vi "CRYWait Graph Close.vi"(10 "vi reference":refnum<vi>) -> ()   [LabVIEW 2013]
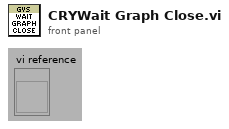
[diagram p1: front panel]
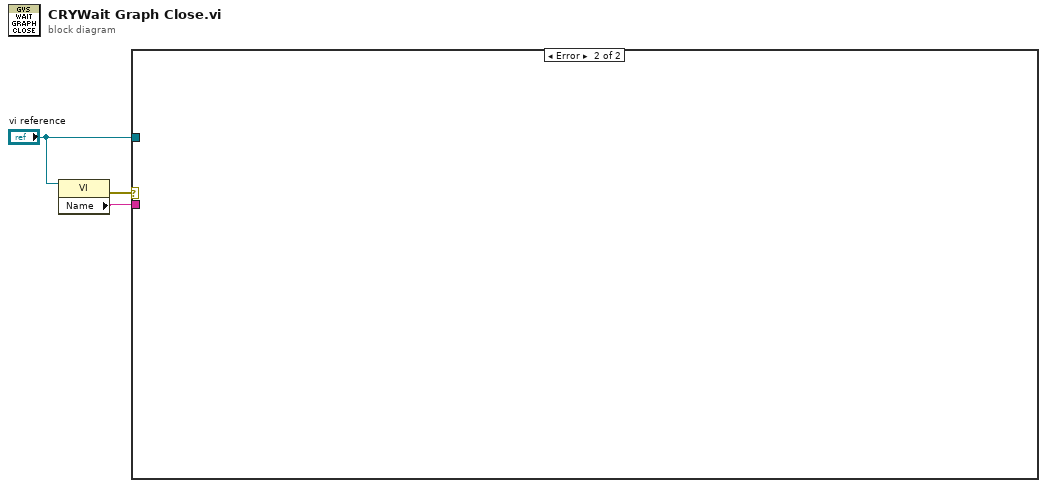
[diagram p0: block diagram]
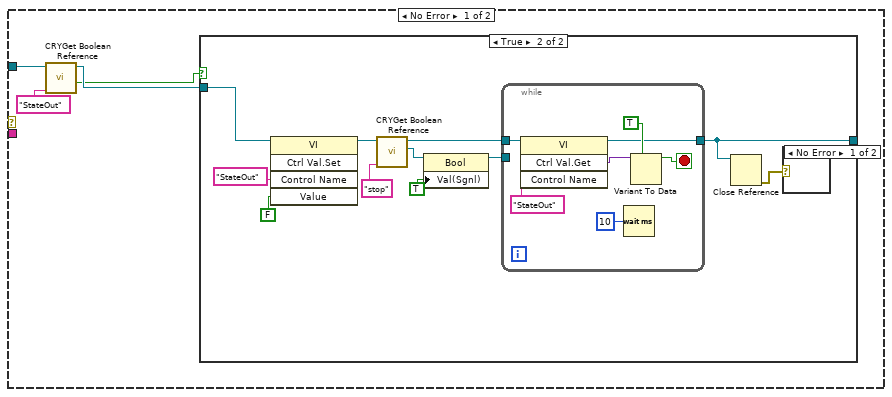
[diagram p2: hidden frame]
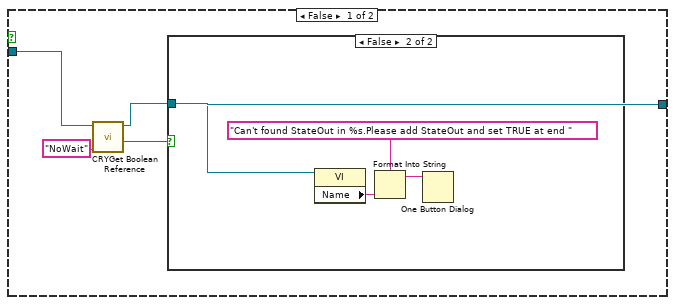
[diagram p3: hidden frame]
diagram:
  n1 = property class="VI"(reference="vi reference") -> (error out=w3:errorcluster, "Name"=w1:string)  [unwired: 1 in, 1 out]
  n2 = case shown="Error" w3 {
    tunnel: "vi reference" -> [w6 _]
    tunnel: w1 -> [_ _]
    frame No Error {
      n3 = call "CRYGet Boolean Reference.vi"("Label Name"="StateOut", "VI Refnum"=w6) -> ("Exist?"=w4:bool, "VI Refnum Out"=w5:refnum<vi>)  [unwired: 7 in, 1 out]
      n4 = case shown="True" w4 {
        tunnel: w5 -> [w10 w19]
        tunnel: [w9 w17] -> _
        frame False {
          n5 = call "CRYGet Boolean Reference.vi"("Label Name"="NoWait", "VI Refnum"=w10) -> ("Exist?"=w8:bool, "VI Refnum Out"=w9:refnum<vi>)  [unwired: 7 in, 1 out]
          n6 = case shown="False" w8 {
            tunnel: w9 -> [_ w12]
            frame True {
            }
            frame False {
              n7 = property class="VI"(reference=w12) -> ("Name"=w14:string)  [unwired: 1 in, 2 out]
              n8 = Format Into String(format string="Can't found StateOut in %s.Please add StateOut and set TRUE at end " ("message"), w14) -> (resulting string=w13:string)  [unwired: 2 in, 1 out]
              n9 = One Button Dialog(message=w13) -> ()  [unwired: 1 in, 1 out]
            }
          }
        }
        frame True {
          n10 = invoke class="VI" method="Ctrl Val.Set"(reference=w19, "Control Name"="StateOut", "Value"=FALSE) -> (reference out=w21:refnum<vi>)  [unwired: 2 in, 4 out]
          n11 = call "CRYGet Boolean Reference.vi"("Label Name"="stop", "VI Refnum"=w21) -> ("Boolean Ref"=w24:refnum<vi>, "VI Refnum Out"=w20:refnum<vi>)  [unwired: 7 in, 1 out]
          n12 = property class="Bool"(reference=w24, "Val(Sgnl)"=TRUE) -> (reference out=w18:refnum<vi>)  [unwired: 1 in, 1 out]
          n13 = while {
            tunnel: w20 -> [w32]
            tunnel: [w28] -> w17
            tunnel: w18 -> [_]
            stop <- w29 stop-if-true
            n14 = invoke class="VI" method="Ctrl Val.Get"(reference=w32, "Control Name"="StateOut") -> (reference out=w28:refnum<vi>, "Get Control Value Variant"=w31:variant)  [unwired: 2 in, 2 out]
            n15 = Wait (ms)(milliseconds to wait=u32 10) -> ()  [unwired: 1 out]
            n16 = Variant To Data(type=TRUE, Variant=w31) -> (data=w29:bool)  [unwired: 1 in, 1 out]
          }
          n17 = Close Reference(reference=w17) -> (error out=w16:errorcluster)  [unwired: 1 in]
          n18 = case shown="No Error" w16 {
            frame No Error {
            }
            frame Error {
            }
          }
        }
      }
    }
    frame Error {
    }
  }
